vi "MeasureData.vi"(8 "error in (no error)":errorcluster, 10 "Process in":refnum<vi>, 11 "SR830 in":refnum<vi>) -> (0 "Error Out":errorcluster, 3 "Process out":refnum<vi>)   [LabVIEW 2016]
uses:
  controls/LockIn.ctl
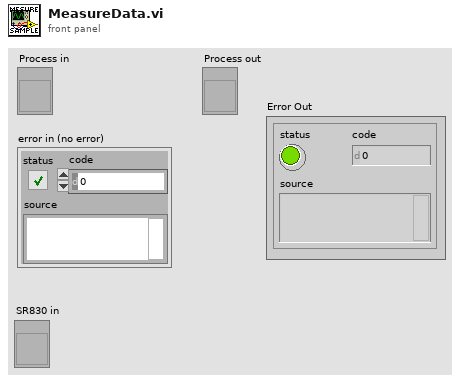
[diagram p1: front panel]
types:
  T1 = typedef "LockIn.ctl" = cluster{"Port":refnum<visa-resource-name>, "Is connected?":bool, "Sensivity Ovld":bool, "lockin-open":bool, "lockin-save":bool, "Reference":cluster{"Source ":u16, "Frequency":dbl}, "Channel Display":cluster{"Channel 1":u16, "Channel 2":u16}, "Sensivity":cluster{"Dynamic Reserve":i16, "Sensitivity":i16, "Time Constant":u16, "Low Pass Filter":u16}, "Display":cluster{"Channel One":dbl, "Channel Two":dbl, "Reference":dbl}, "Parameter Values":cluster{"X-Value":dbl, "Y-Value":dbl, "R-Value":dbl, "Theta-Value":dbl, "Aux In 1 Value":dbl, "Aux In 2 Value":dbl, "Aux In 3 Value":dbl, "Aux In 4 Value":dbl, "Reference Frequency":dbl, "Channel 1 Display":dbl, "Channel 2 Display":dbl}}
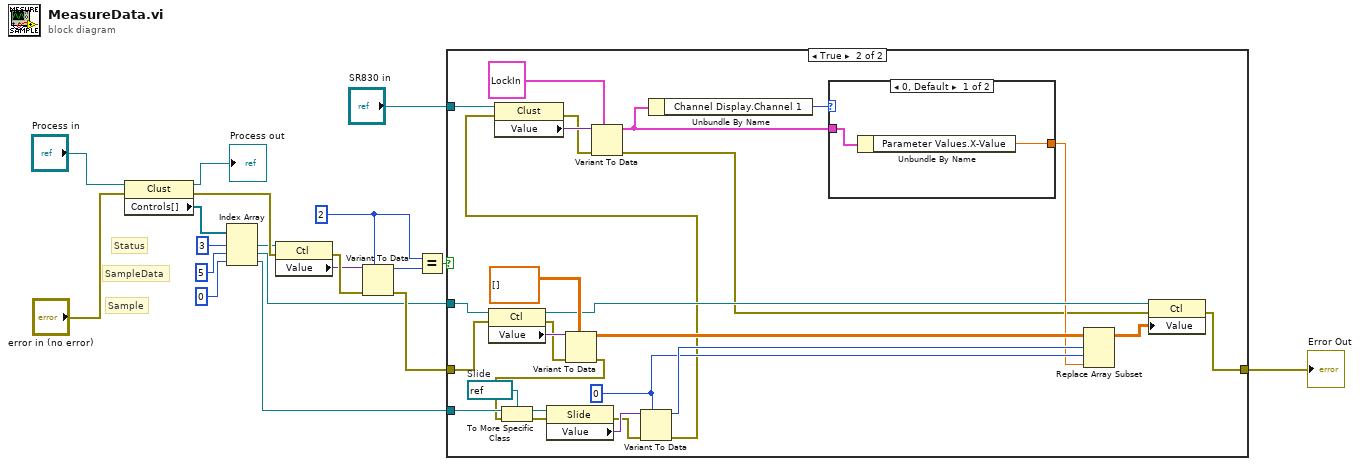
[diagram p0: block diagram]
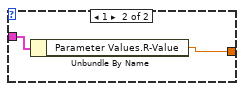
[diagram p3: hidden frame]
diagram:
  w15 = 2
  # "Sample"
  # "SampleData"
  # "Status"
  n1 = property class="Clust"(reference="Process in", error in="error in (no error)") -> (reference out=→"Process out":refnum<vi>, error out=w11:errorcluster, "Controls[]"=w8:refnum<vi>[])
  n2 = Index Array(array=w8, index #1=3 ("index"), index #2=5 ("index"), index #3=0 ("index")) -> (element #1=w10:refnum<vi>, element #2=w6:refnum<vi>, element #3=w4:refnum<vi>)
  n3 = property class="Ctl"(reference=w10, error in=w11) -> (error out=w13:errorcluster, "Value"=w12:variant)  [unwired: 1 out]
  n4 = Variant To Data(error in=w13, type=w15, Variant=w12) -> (data=w14:i32, error out=w17:errorcluster)
  n5 = Equal?(x=w15, y=w14) -> (x = y?=w16:bool)
  n6 = case shown="True" w16 {
    tunnel: w17 -> [w20 w46]
    tunnel: [w20 w33] -> w3
    tunnel: w6 -> [_ w47]
    tunnel: w4 -> [_ w41]
    tunnel: "SR830 in" -> [_ w30]
    frame False {
    }
    frame True {
      w31 = 0
      w40 = refnum<vi> refnum  # Slide
      n7 = property class="Ctl"(reference=w47, error in=w46) -> (reference out=w34:refnum<vi>, error out=w44:errorcluster, "Value"=w45:variant)
      n8 = Variant To Data(error in=w44, type=dbl[][] [], Variant=w45) -> (data=w42:dbl[][], error out=w38:errorcluster)
      n9 = To More Specific Class(target class=w40, reference=w41, error in=w38) -> (specific class reference=w39:refnum<vi>, error out=w37:errorcluster)
      n10 = property class="Slide"(reference=w39, error in=w37) -> (error out=w35:errorcluster, "Value"=w36:variant)  [unwired: 1 out]
      n11 = Variant To Data(error in=w35, type=w31, Variant=w36) -> (data=w32:i32, error out=w26:errorcluster)
      n12 = property class="Clust"(reference=w30, error in=w26) -> (error out=w28:errorcluster, "Value"=w29:variant)  [unwired: 1 out]
      n13 = Variant To Data(error in=w28, type=T1 {"Port"="", "Is connected?"=FALSE, "Sensivity Ovld"=FALSE, "lockin-open"=FALSE, "lockin-save"=FALSE, "Reference"={"Source "=0, "Frequency"=1000.0}, "Channel Display"={"Channel 1"=1, "Channel 2"=1}, "Sensivity"={"Dynamic Reserve"=0, "Sensitivity"=25, "Time Constant"=11, "Low Pass Filter"=2}, "Display"={"Channel One"=0.0, "Channel Two"=0.0, "Reference"=0.0}, "Parameter Values"={"X-Value"=0.4395283849063103, "Y-Value"=0.15216351416612506, "R-Value"=0.4452242651211462, "Theta-Value"=0.7740615187954734, "Aux In 1 Value"=0.06531541538388264, "Aux In 2 Value"=0.3838864256017631, "Aux In 3 Value"=0.5316030093003845, "Aux In 4 Value"=0.8022202949601139, "Reference Frequency"=0.45644404910704495, "Channel 1 Display"=0.9592975044755206, "Channel 2 Display"=0.7364994800777196}} ("Lock-In-Amplifier"), Variant=w29) -> (data=w23:T1, error out=w21:errorcluster)
      n14 = Unbundle By Name(w23) -> ("Channel Display.Channel 1"=w24:u16)
      n15 = case shown="0, Default" w24 {
        tunnel: w23 -> [w49 w51]
        tunnel: [w48 w50] -> w22
        frame 0, Default {
          n16 = Unbundle By Name(w49) -> ("Parameter Values.X-Value"=w48:dbl)
        }
        frame 1 {
          n17 = Unbundle By Name(w51) -> ("Parameter Values.R-Value"=w50:dbl)
        }
      }
      n18 = Replace Array Subset(array=w42, new element=w22, index (row)=w32, index (col)=w31) -> (w25:dbl[][])
      n19 = property class="Ctl"(reference=w34, error in=w21, "Value"=w25) -> (error out=w33:errorcluster)  [unwired: 1 out]
    }
  }
  "Error Out" <- w3
